vi "fractional to uint8.vi"(11 "x":dbl format="%#_13g") -> (3 "U8 number":u8 format="%08b")   [LabVIEW 2017]
uses:
  <vilib>/imath/engines/lvmath2/RunTimeEngine/Managers/WorkSpace/UID Generator.vi
  <vilib>/imath/engines/lvmath2/RunTimeEngine/RangeToken/NIMS_Range_R2 - Integer.vi
  <instcachedir>/0/NIMS_Range_R2 - Integer_C9C65F8E5BDB44CDAB4330270A9F1B77.lvgen/NIMS_Range_R2 - Integer_C9C65F8E5BDB44CDAB4330270A9F1B77_000.vi
  <vilib>/imath/engines/lvmath2/RunTimeEngine/CommandStatement/MC_CommandStatement_break.vi
  <vilib>/imath/engines/lvmath2/RunTimeEngine/RowToken/NIMS_RowToken_M_SorRV.vi
  <instcachedir>/0/NIMS_RowToken_M_SorRV_21F1FB7AB8754AE585ABEB817147FA69.lvgen/NIMS_RowToken_M_SorRV_21F1FB7AB8754AE585ABEB817147FA69_001.vi
  <vilib>/imathl/engines/lvmath/Functions/Error Handling/Create Error.vi
  <vilib>/imath/engines/lvmath2/RunTimeEngine/RunTimeType/NIMS_RunTimeType_From StrictType (excl LVString).vi
  <instcachedir>/0/NIMS_RunTimeType_From StrictType (excl LVString)_DC56D72BB6B948F98D63F1A957D87C42.lvgen/NIMS_RunTimeType_From StrictType (excl LVString)_DC56D72BB6B948F98D63F1A957D87C42_000.vi
  <vilib>/imath/engines/lvmath2/RunTimeEngine/LocalVariableDefStatement/MC_LocalVariableDefStatement_Display.vi
  <vilib>/imath/engines/lvmath2/RunTimeEngine/BuiltInFunctions/length/NIMS_length(GM).vi
  <instcachedir>/0/NIMS_length(GM)_47CEC356FCE0482D9BA47DC61C99F2C7.lvgen/NIMS_length(GM)_47CEC356FCE0482D9BA47DC61C99F2C7_001.vi
  <vilib>/imath/engines/lvmath2/RunTimeEngine/IndexRead/NIMS M(S).vi
  <instcachedir>/0/NIMS M(S)_B826C018497E4940AE96BD27B540B6FB.lvgen/NIMS M(S)_B826C018497E4940AE96BD27B540B6FB_005.vi
  <vilib>/imath/engines/lvmath2/RunTimeEngine/Managers/SymbolTable/Clear UID.vi
  <vilib>/imath/engines/lvmath2/RunTimeEngine/NodeEndStatement/NIMS_NodeEndStatement_Output.vi
  <instcachedir>/0/NIMS_NodeEndStatement_Output_53EC0D466D134D7ABD903AC30B43404B.lvgen/NIMS_NodeEndStatement_Output_53EC0D466D134D7ABD903AC30B43404B_012.vi
  <instcachedir>/0/NIMS_NodeEndStatement_Output_53EC0D466D134D7ABD903AC30B43404B.lvgen/NIMS_NodeEndStatement_Output_53EC0D466D134D7ABD903AC30B43404B_001.vi
  <vilib>/imath/engines/lvmath2/RunTimeEngine/ErrorHandling/NIMS_Finalize Error.vi
  <vilib>/imath/engines/lvmath2/RunTimeEngine/Managers/SymbolTable/NIMS_WorkSpace.lvlib
panel:
  out "Array":bool[](array[boolean])
  out "output":dbl format="%#_6f"
  out "x_binary":i32[][](array[numeric])
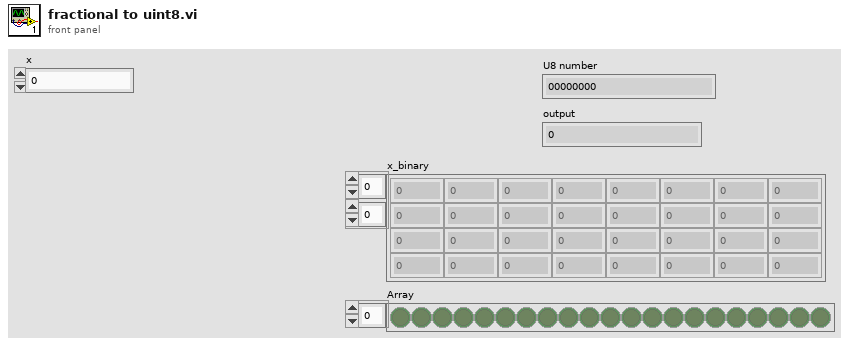
[diagram p1: front panel]
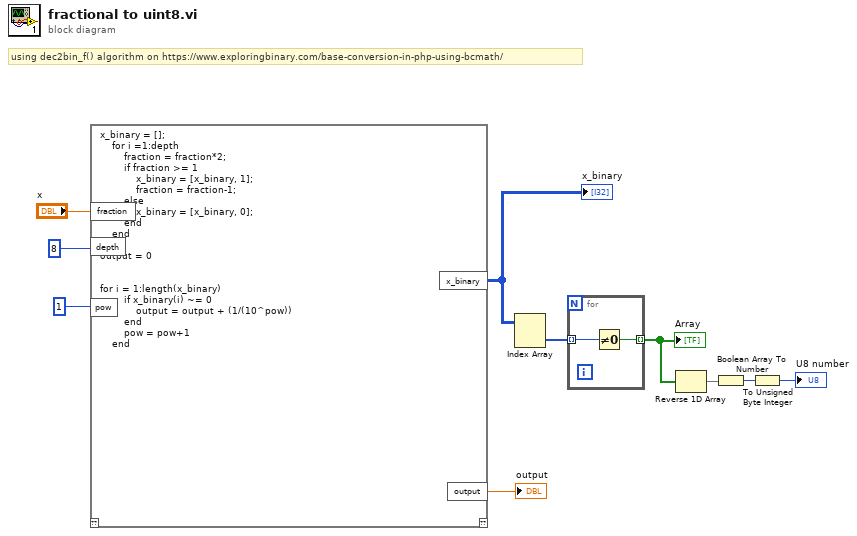
[diagram p0: block diagram]
diagram:
  # "using dec2bin_f() algorithm on https://www.exploringbinary.com/base-conversion-in-php-using-bcmath/"
  n1 = mathscript code="x_binary = [];\n    for i =1:depth    \n        fraction = fraction*2;\n        if fraction >= 1\n            x_binary = [x_binary, 1];\n            fraction = fraction-1;\n        else\n            x_binary = [x_binary, 0];\n        end        \n    end\n\noutput = 0\n\n\nfor i = 1:length(x_binary)\n        if x_binary(i) ~= 0\n            output = output + (1/(10^pow))\n        end\n        pow = pow+1\n    end"("fraction"="x", "depth"=8, "pow"=1) -> ("x_binary"=w6:i32[][], "output"=→"output":dbl)  [unwired: 1 in, 1 out]
  "x_binary" <- w6
  n2 = Index Array(array=w6) -> (element=w5:i32[])  [unwired: 2 in]
  n3 = for {
    tunnel: w5 -> [w12] mode=indexing
    tunnel: [w11] -> w4 mode=indexing
    n4 = Not Equal To 0?(x=w12) -> (x != 0?=w11:bool)
  }
  "Array" <- w4
  n5 = Reverse 1D Array(array=w4) -> (reversed array=w3:bool[])
  n6 = Boolean Array To Number(Boolean array=w3) -> (number=w1:u32)
  n7 = To Unsigned Byte Integer(number=w1) -> (unsigned 8bit integer=→"U8 number":u8)
